vi "Upload.vi"   [LabVIEW 2012]
uses:
  <vilib>/addons/database/Auxilliary.llb/DB Tools DataTypes.ctl
  <vilib>/addons/database/Auxilliary.llb/DB Tools Parameter Dir.ctl
  <vilib>/addons/database/NI_Database_API.lvlib
types:
  T1 = typedef "NI_Database_API.lvlib/DB Tools DataTypes.ctl" = enum16{"String", "Long (I32)", "Single (SGL)", "Double (DBL)", "Date/Time", "Binary"}
  T2 = typedef "NI_Database_API.lvlib/DB Tools Parameter Dir.ctl" = enum32{"Input", "Output", "Input/Output", "Return Value"}
  T3 = cluster{"userCode":string, "userName":string, "userStatus":string, "connectionMode":string, "takesTime":string, "countDone":string, "countOK":string, "countNG":string, "rigStatus":string, "productsName":string, "partCode1":string, "partCode2":string, "partCode3":string}
  T4 = cluster{"parameter name":string, "type":T1, "direction":T2, "partCode3":string}
  T5 = cluster{"parameter name":string, "type":T1, "direction":T2, "Variant":variant}
  T6 = cluster{"parameter name":string, "type":T1, "direction":T2, "parameter name":string}
  T7 = cluster{"parameter name":string, "type":T1, "direction":T2, "Variant":variant}[]
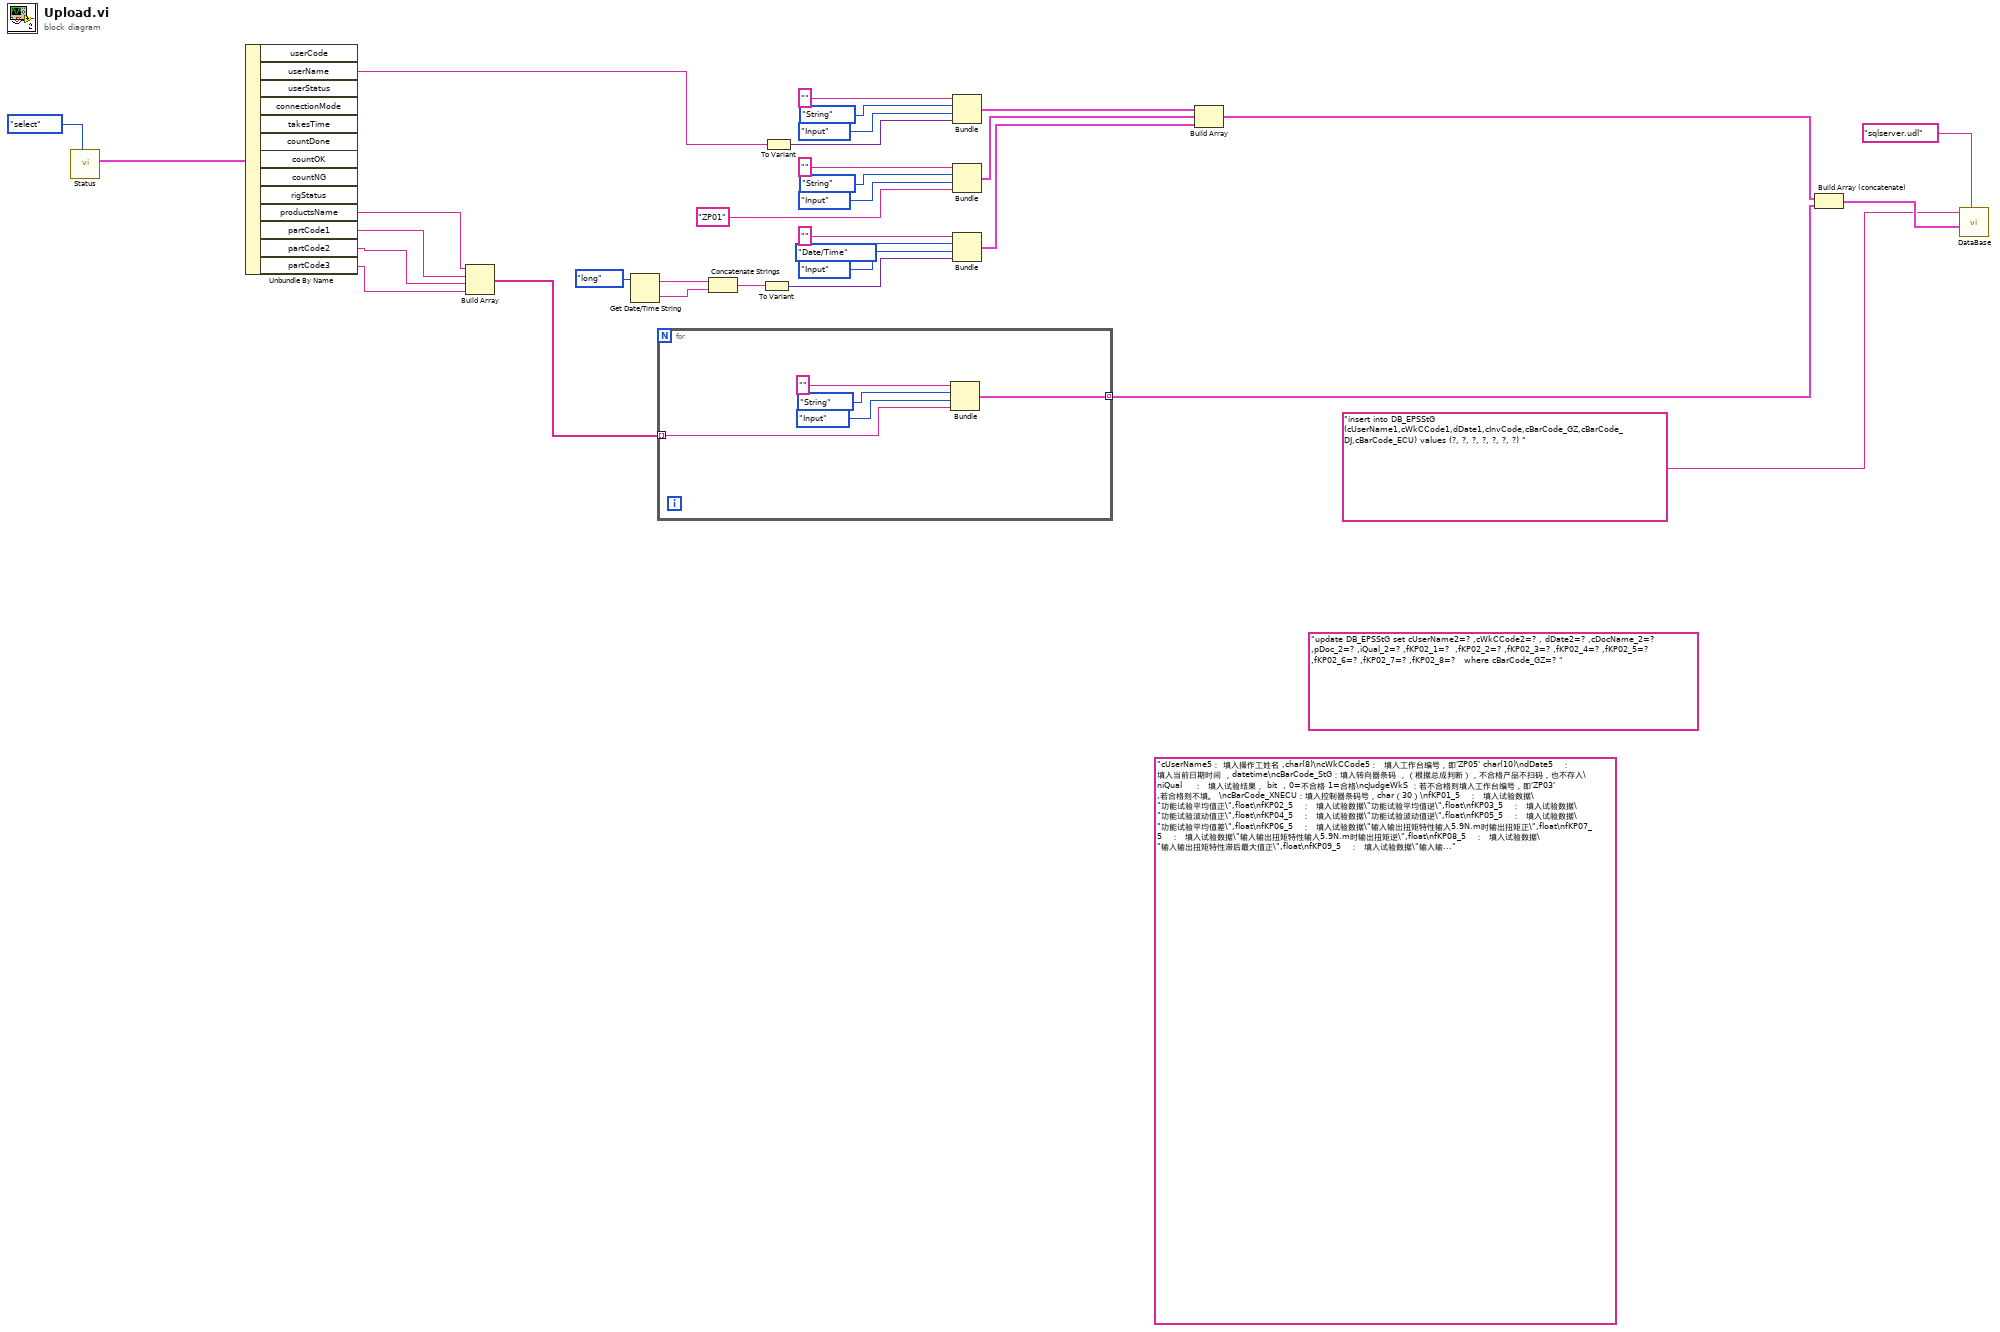
[diagram p0: block diagram]
diagram:
  (unwired) "update DB_EPSStG set cUserName2=? ,cWkCCode2=? , dDate2=? ,cDocName_2=? ,pDoc_2=? ,iQual_2=? ,fKP02_1=?  ,fKP02_2=? ,fKP02_3=? ,fKP02_4=? ,fKP02_5=? ,fKP02_6=? ,fKP02_7=? ,fKP02_8=?   where cBarCode_GZ=? " ("SQL query")
  (unwired) "cUserName5： 填入操作工姓名 ,char(8)\ncWkCCode5：  填入工作台编号，即'ZP05' char(10)\ndDate5   ：  填入当前日期时间 ，datetime\ncBarCode_StG：填入转向器条码 ，（根据总成判断），不合格产品不扫码，也不存入\niQual    ：  填入试验结果， bit  , 0=不合格 1=合格\ncJudgeWkS ：若不合格则填入工作台编号，即'ZP03' ,若合格则不填。 \ncBarCode_XNECU：填入控制器条码号，char（30）\nfKP01_5   ：  填入试验数据\"功能试验平均值正\",float\nfKP02_5   ：  填入试验数据\"功能试验平均值逆\",float\nfKP03_5   ：  填入试验数据\"功能试验波动值正\",float\nfKP04_5   ：  填入试验数据\"功能试验波动值逆\",float\nfKP05_5   ：  填入试验数据\"功能试验平均值差\",float\nfKP06_5   ：  填入试验数据\"输入输出扭矩特性输入5.9N.m时输出扭矩正\",float\nfKP07_5   ：  填入试验数据\"输入输出扭矩特性输入5.9N.m时输出扭矩逆\",float\nfKP08_5   ：  填入试验数据\"输入输出扭矩特性滞后最大值正\",float\nfKP09_5   ：  填入试验数据\"输入输出扭矩特性滞后最大值逆\",float\nfKP10_5   ：  填入试验数据\"输入输出扭矩特性对称度\",float\nfKP11_5   ：  填入试验数据\"扭矩传感器特性滞后最大值正\",float\nfKP12_5   ：  填入试验数据\"扭矩传感器特性滞后最大值逆\",float\nfKP13_5   ：  填入试验数据\"扭矩传感器特性对称度\",float\nfKP14_5   ：  填入试验数据\"空载平均值正\",float\nfKP15_5   ：  填入试验数据\"空载平均值逆\",float\nfKP16_5   ：  填入试验数据\"空载平均值差\",float\nfKP17_5   ：  填入试验数据\"空载波动值正\",float\nfKP18_5   ：  填入试验数据\"空载波动值逆\",float\nfKP19_5   ：  填入试验数据\"空载最大值正\",float\nfKP20_5   ：  填入试验数据\"空载最大值逆\",float\n\ncDocName_5：  填入试验报告文件名称，char（40），根据实际文件名，可与本机存储的文件名相同。\npDoc_5    ：  写入试验报告， image ,  实际的试验报告文件 \n     iQual_5   ：  填入试验结果， bit  , 0=不合格 1=合格\n" ("SQL query")
  n1 = call "Status.vi"("模式"=enum16{"select", "insert", "update", "delete"}."select") -> ("元素"=w10:T3)  [unwired: 10 in]
  n2 = Unbundle By Name(w10) -> ("userName"=w9:string, "productsName"=w7:string, "partCode1"=w6:string, "partCode2"=w5:string, "partCode3"=w4:string)  [unwired: 8 out]
  n3 = Build Array(w7, w6, w5, w4) -> (w3:string[])
  n4 = Get Date/Time String ("获取日期/时间字符串")(date format (0)=enum16{"short", "long", "abbreviated"}."long" ("日期格式(0)")) -> (date string=w14:string, time string=w15:string)  [unwired: 2 in]
  n5 = for {
    tunnel: w3 -> [w34] mode=indexing
    tunnel: [w33] -> w2 mode=indexing
    n6 = Bundle("parameter name"="", "type"=DB_Tools_DataTypes."String", "direction"=DB_Tools_Parameter_Dir."Input", "partCode3"=w34) -> (w33:T4)  [unwired: 1 in]
  }
  n7 = Concatenate Strings(w14, w15) -> (w13:string)
  n8 = To Variant(anything=w13) -> (Variant=w18:variant)
  n9 = To Variant(anything=w9) -> (Variant=w17:variant)
  n10 = Bundle("parameter name"="", "type"=DB_Tools_DataTypes."String", "direction"=DB_Tools_Parameter_Dir."Input", "Variant"=w17) -> (w28:T5)  [unwired: 1 in]
  n11 = Bundle("parameter name"="", "type"=DB_Tools_DataTypes."String", "direction"=DB_Tools_Parameter_Dir."Input", "parameter name"="ZP01") -> (w20:T6)  [unwired: 1 in]
  n12 = Bundle("parameter name"="", "type"=DB_Tools_DataTypes."Date/Time", "direction"=DB_Tools_Parameter_Dir."Input", "Variant"=w18) -> (w19:T5)  [unwired: 1 in]
  n13 = Build Array(w28, w20, w19) -> (w8:T7)
  n14 = Build Array (concatenate)(w8, w2) -> (w12:T7)
  n15 = call "DataBase.vi"("udl名称"="sqlserver.udl", "parameters"=w12, "SQL query"="insert into DB_EPSStG (cUserName1,cWkCCode1,dDate1,cInvCode,cBarCode_GZ,cBarCode_DJ,cBarCode_ECU) values (?, ?, ?, ?, ?, ?, ?) ") -> ()  [unwired: 8 in, 1 out]
